vi "Manipulator Controller Global.vi"() -> ()   [LabVIEW 2018]
panel:
  in  "Manipulator Right Trigger":dbl
  in  "Manipulator Left Trigger":dbl
  in  "Manipulator Right Stick Y":dbl
  in  "Manipulator Right Stick X":dbl
  in  "Manipulator Left Stick Y":dbl
  in  "Manipulator Left Stick X":dbl
  out "Manipulator Right Start":bool
  out "Manipulator Left Start":bool
  out "Manipulator Right Bumper":bool
  out "Manipulator Left Bumper":bool
  out "Manipulator Button Y":bool
  out "Manipulator Button X":bool
  out "Manipulator Button B":bool
  out "Manipulator Button A":bool
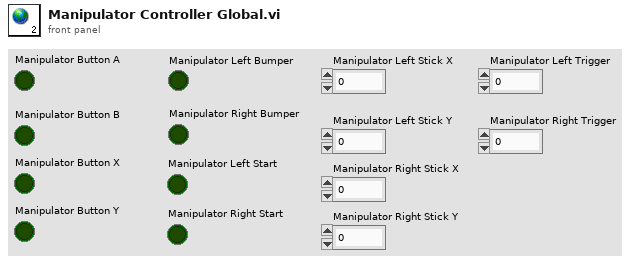
[diagram p1: front panel]
diagram:
